vi "Init.vi"(8 "error in (no error)":errorcluster, 11 "LHL Actor in":refnum<class "LHL Actor.lvclass">) -> (0 "error out":errorcluster, 3 "LHL Actor out":refnum<class "LHL Actor.lvclass">)   [LabVIEW 2020, in "LHL Actor.lvlib" / "LHL Actor.lvclass"]
uses:
  LHL Actor.lvclass
  LHL Actor.lvclass/LHL Actor.ctl
  <vilib>/Utility/config.llb/Read Key (String).vi
  <vilib>/Utility/config.llb/NI_LVConfig.lvlib
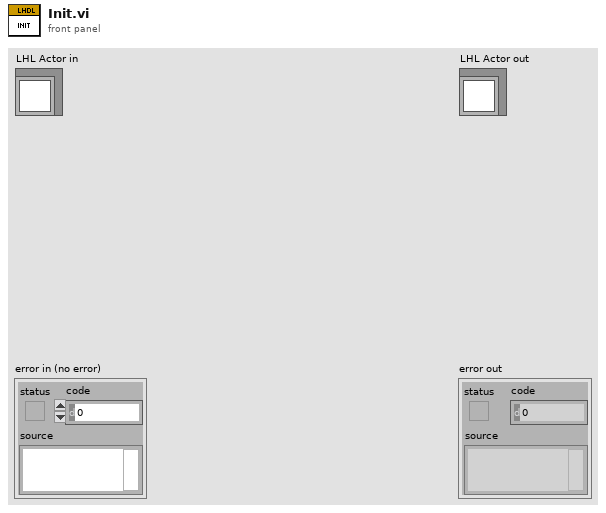
[diagram p1: front panel]
types:
  T1 = typedef "NI_LVConfig.lvlib/Config Data RefNum.ctl" = refnum<k1>
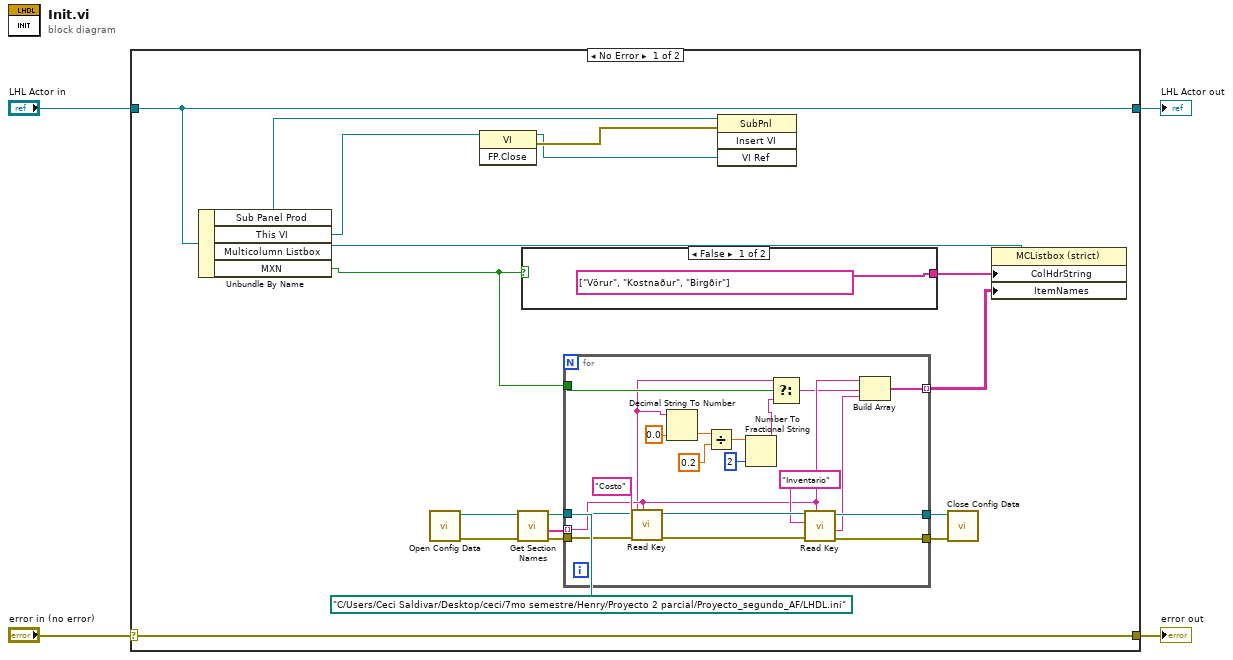
[diagram p0: block diagram]
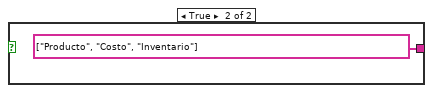
[diagram p2: hidden frame]
diagram:
  n1 = case shown="No Error" "error in (no error)" {
    selector: "error in (no error)" -> [w22 w46]
    tunnel: [w22 w46] -> w3
    tunnel: [w17 w45] -> w1
    tunnel: "LHL Actor in" -> [w17 w45]
    frame No Error {
      n2 = Unbundle By Name(w17) -> ("Sub Panel Prod"=w18:refnum<vi>, "This VI"=w19:refnum<vi>, "Multicolumn Listbox"=w16:refnum<vi>, "MXN"=w5:bool)
      n3 = call <vilib>:"Open Config Data.vi"("configuration file path"=path "C:/Users/Ceci Saldivar/Desktop/ceci/7mo semestre/Henry/Proyecto 2 parcial/Proyecto_segundo_AF/LHDL.ini") -> ("error out"=w10:errorcluster, "refnum"=w13:T1)  [unwired: 8 in, 1 out]
      n4 = invoke class="VI" method="FP.Close"(reference=w19) -> (reference out=w20:refnum<vi>, error out=w21:errorcluster)  [unwired: 2 in, 1 out]
      n5 = call <vilib>:"Get Section Names.vi"("error in (no error)"=w10, "refnum"=w13) -> ("error out"=w9:errorcluster, "section names"=w12:string[], "refnum out"=w11:T1)  [unwired: 7 in]
      n6 = case shown="False" w5 {
        tunnel: [string[] ["Vörur", "Kostnaður", "Birgðir"] ("Column Header Strings[]") string[] ["Producto", "Costo", "Inventario"] ("Column Header Strings[]")] -> w15
        frame False {
        }
        frame True {
        }
      }
      n7 = for {
        tunnel: w12 -> [w36] mode=indexing
        tunnel: w11 -> [w43]
        tunnel: w9 -> [w42]
        tunnel: [w38] -> w6
        tunnel: [w37] -> w7
        tunnel: [w34] -> w8 mode=indexing
        tunnel: w5 -> [w33]
        n8 = call-poly <vilib>:"Read Key.vi"("section"=w36, "error in (no error)"=w42, "key"="Costo", "refnum"=w43) -> ("error out"=w39:errorcluster, "value"=w27:string, "refnum out"=w41:T1)  [unwired: 4 in, 1 out]
        n9 = Decimal String To Number(string=w27, default (0L)=0.0) -> (number=w31:dbl)  [unwired: 1 in, 1 out]
        n10 = Divide(x=w31, y=0.2) -> (x/y=w29:dbl)
        n11 = Number To Fractional String(number=w29, precision (6)=i16 2) -> (F-format string=w26:string)  [unwired: 2 in]
        n12 = Select(t=w27, s=w33, f=w26) -> (s? t:f=w25:string)
        n13 = call-poly <vilib>:"Read Key.vi"("section"=w36, "error in (no error)"=w39, "key"="Inventario", "refnum"=w41) -> ("error out"=w37:errorcluster, "value"=w35:string, "refnum out"=w38:T1)  [unwired: 4 in, 1 out]
        n14 = Build Array(w36, w25, w35) -> (w34:string[])
      }
      n15 = invoke class="SubPnl" method="Insert VI"(reference=w18, error in=w21, "VI Ref"=w20) -> ()  [unwired: 1 in, 4 out]
      n16 = call <vilib>:"Close Config Data.vi"("error in (no error)"=w7, "refnum"=w6) -> ()  [unwired: 8 in, 2 out]
      n17 = property class="MCListbox (strict)"(reference=w16, "ColHdrString"=w15, "ItemNames"=w8) -> ()  [unwired: 1 in, 2 out]
    }
    frame Error {
    }
  }
  "error out" <- w3
  "LHL Actor out" <- w1
